vi "根据棋子图片获得信息.vi"(0 "棋子":u16(ring)) -> (1 "棋子类型":enum16{"士兵", "骑士", "主教", "战车", "皇后", "国王", "空"}(ring), 2 "背景颜色":enum16{"白色", "绿色"}(ring), 3 "棋子颜色":enum16{"银色", "黑色"}(ring))   [LabVIEW 2017]
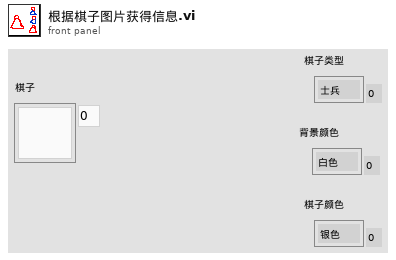
[diagram p1: front panel]
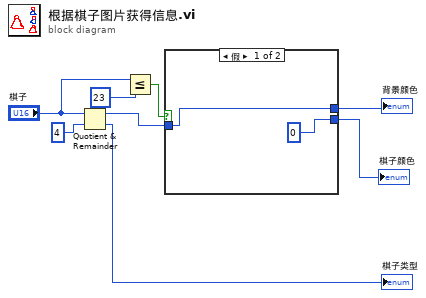
[diagram p0: block diagram]
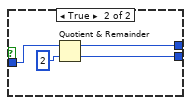
[diagram p2: hidden frame]
diagram:
  n1 = Quotient & Remainder(x="棋子", y=u16 4) -> (x-y*floor(x/y)=w3:u16, floor(x/y)=→"棋子类型":u16)
  n2 = Less Or Equal?(x="棋子", y=u16 23) -> (x <= y?=w6:bool)
  n3 = case shown="假" w6 {
    tunnel: w3 -> [w10 w14]
    tunnel: [u16 0 w12] -> w2
    tunnel: [w10 w11] -> w1
    frame False {
    }
    frame True {
      n4 = Quotient & Remainder(x=w14, y=u16 2) -> (x-y*floor(x/y)=w11:u16, floor(x/y)=w12:u16)
    }
  }
  "棋子颜色" <- w2
  "背景颜色" <- w1
